vi "Add Modbus Addr (Grp).vi"(8 "error in":errorcluster, 9 "Starting Address (SGL)":i32, 11 "ChanGrp.lvclass":refnum<class "ChanGrp.lvclass">) -> (0 "error our":errorcluster, 1 "Next Address (SGL)":i32, 3 "ChanGrp.lvclass":refnum<class "ChanGrp.lvclass">)   [LabVIEW 2012, in "Configuration Grandmaster.lvlib" / "ChanGrp.lvclass"]
uses:
  ChanGrp.lvclass
  ChanGrp.lvclass/ChanGrp.ctl
  Measurements/Class Channel/Channel.lvclass
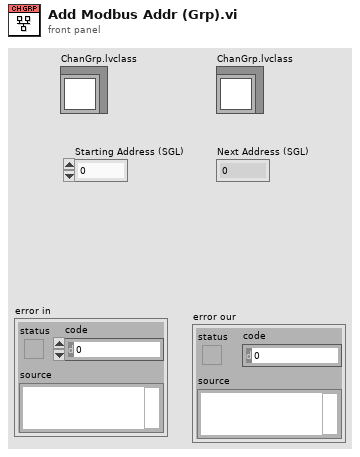
[diagram p1: front panel]
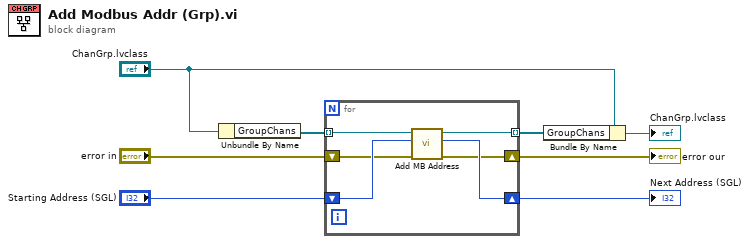
[diagram p0: block diagram]
diagram:
  n1 = Unbundle By Name("ChanGrp.lvclass") -> ("GroupChans"=w5:refnum<class "Channel.lvclass">[])
  n2 = for {
    tunnel: w5 -> [w12] mode=indexing
    tunnel: [w11] -> w6 mode=indexing
    shift-right: [w14] -> w8
    shift-left: "Starting Address (SGL)" -> [w13]
    shift-right: [w10] -> w1
    shift-left: "error in" -> [w9]
    n3 = call "Add MB Address.vi"("error in (no error)"=w9, "Starting Address (SGL) in"=w13, "Channel in"=w12) -> ("error out"=w10:errorcluster, "Next Address (SGL)"=w14:i32, "Channel out"=w11:refnum<class "Channel.lvclass">)  [unwired: 6 in]
  }
  "Next Address (SGL)" <- w8
  "error our" <- w1
  n4 = Bundle By Name(cluster="ChanGrp.lvclass", "GroupChans"=w6) -> (→"ChanGrp.lvclass":refnum<class "ChanGrp.lvclass">)
